vi "RSZVB Trace Shift Response Value.vi"(4 "Magnitude (0.0 dB)":dbl format="%^.3e", 5 "Imaginary (0.0)":dbl format="%^.3e", 6 "Real (0.0)":dbl format="%^.3e", 7 "Phase (0.0 deg)":dbl format="%^.3e", 8 "error in (no error)":errorcluster {"code" format="%.0x"}, 9 "Window (Trace) (1)":i32=1, 10 "Window (1)":i32=1, 11 "VISA session":refnum<visa-resource-name>) -> (0 "error out":errorcluster {"code" format="%.0x"}, 3 "dup VISA session":refnum<visa-resource-name>)   [LabVIEW 2011]
doc: "This VI modifies all points of the trace <WndTr> by means of an added and/or a multiplied complex constant. The response values M of the trace are transformed according to:\n\nM_new = M_old * 10^(<Magnitude> / 20dB) * a * e^(j <Phase> / 180Deg) + <Real> + j <Imaginary>\n\nNote(s):\n\n(1) Window:\nNumber of an existing diagram area (defined by means of DISPlay:WINDow<Wnd>:STATe ON).\n\n(2) Window (Trace):\nExisting trace number, assigned by means of DISPlay:WINDow<Wnd>:TRACe<WndTr>:FEED.\n\nRemote-control command(s):\nDISPlay:WINDow<Wnd>:TRACe<WndTr>:Y:OFFSet <Magnitude>[,<Phase>, <Real>, <Imaginary>]"
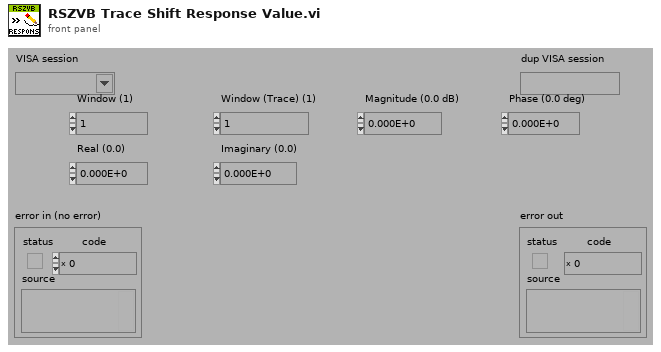
[diagram p1: front panel]
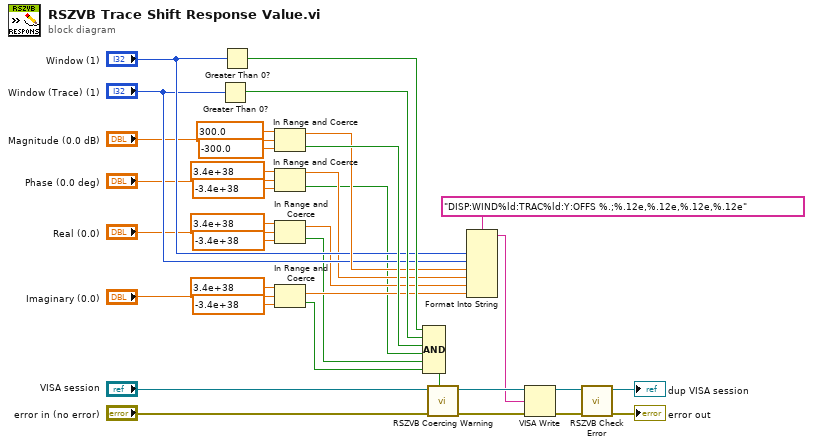
[diagram p0: block diagram]
diagram:
  n1 = Greater Than 0?(x="Window (Trace) (1)") -> (x > 0?=w24:bool)
  n2 = Greater Than 0?(x="Window (1)") -> (x > 0?=w28:bool)
  n3 = In Range and Coerce(upper limit=300.0, x="Magnitude (0.0 dB)", lower limit=-300.0) -> (coerced(x)=w23:dbl, In Range?=w26:bool)
  n4 = In Range and Coerce(upper limit=3.4e+38, x="Phase (0.0 deg)", lower limit=-3.4e+38) -> (coerced(x)=w6:dbl, In Range?=w3:bool)
  n5 = In Range and Coerce(upper limit=3.4e+38, x="Real (0.0)", lower limit=-3.4e+38) -> (coerced(x)=w5:dbl, In Range?=w2:bool)
  n6 = In Range and Coerce(upper limit=3.4e+38, x="Imaginary (0.0)", lower limit=-3.4e+38) -> (coerced(x)=w4:dbl, In Range?=w1:bool)
  n7 = Compound Arithmetic op=AND(w28, w24, w26, w3, w2, w1) -> (w27:bool)
  n8 = call "RSZVB Coercing Warning.vi"("In Range?"=w27, "error in (no error)"="error in (no error)", "VISA session"="VISA session") -> ("error out"=w34:errorcluster, "dup VISA session"=w35:refnum<visa-resource-name>)  [unwired: 7 in]
  n9 = Format Into String(format string="DISP:WIND%ld:TRAC%ld:Y:OFFS %.;%.12e,%.12e,%.12e,%.12e", "Window (1)", "Window (Trace) (1)", w23, w6, w5, w4) -> (resulting string=w25:string)  [unwired: 2 in, 1 out]
  n10 = VISA Write(VISA resource name=w35, write buffer=w25, error in (no error)=w34) -> (VISA resource name out=w32:refnum<visa-resource-name>, error out=w33:errorcluster)  [unwired: 1 out]
  n11 = call "RSZVB Check Error.vi"("error in (no error)"=w33, "VISA session"=w32) -> ("error out"=→"error out":errorcluster, "dup VISA session"=→"dup VISA session":refnum<visa-resource-name>)  [unwired: 8 in]
